vi "CastArrayDependenciesToClusterOrClass.vi"(7 "Dependency Type (Class|Cluster)":variant, 8 "error in (no error)":errorcluster, 10 "index (-1: from start)":i32=-1, 11 "[Dependencies]":refnum<class>[](array[class])) -> (0 "error out":errorcluster, 3 "Dependencies output":variant)   [LabVIEW 2019, in "SMO.lvclass"]
doc: "JKI State Machine Objects (SMO) 1.3.0.56\nJKI - JKI\nCopyright (c) 2017, JKI"
uses:
  SMO.lvclass
  <vilib>/Utility/VariantDataType/Type.ctl
  <vilib>/Utility/VariantDataType/VariantType.lvlib
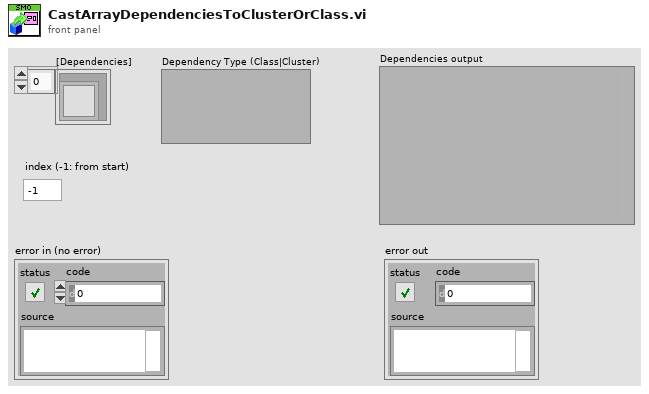
[diagram p1: front panel]
types:
  T1 = typedef "VariantType.lvlib/Type.ctl" = enum8{"Invalid Type", "Void", "I8", "I16", "I32", "I64", "U8", "U16", "U32", "U64", "Single Float", "Double Float", "Extended Float", "Single Complex", "Double Complex", "Extended Complex", "Enum U8", "Enum U16", "Enum U32", "Enum U64", "Single Float With Unit", "Double Float With Unit", "Extended Float With Unit", "Single Complex with Unit", "Double Complex with Unit", "Extended Complex with Unit", "Boolean", "String", "Path", "Picture", "Tag", "Array", "Cluster", "Variant", "LV Variant", "Waveform", "Timestamp", "Digital Waveform", "Digital Data", "ExpressData", "Refnum", "External Data", "VI", "Poly VI", "LabVIEW Class Instance", "Fixed Point"}
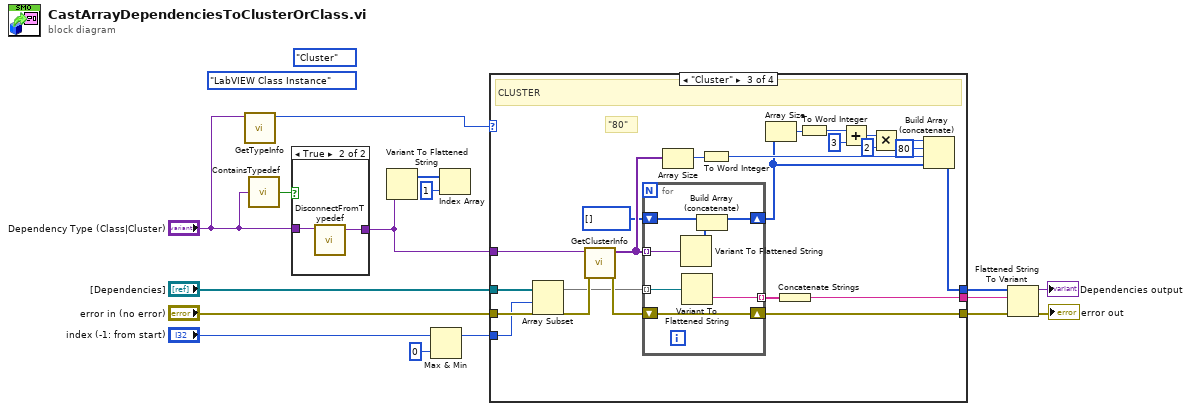
[diagram p0: block diagram]
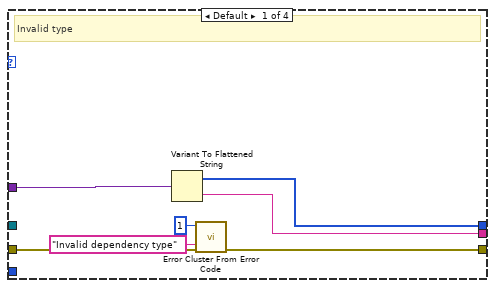
[diagram p3: hidden frame]
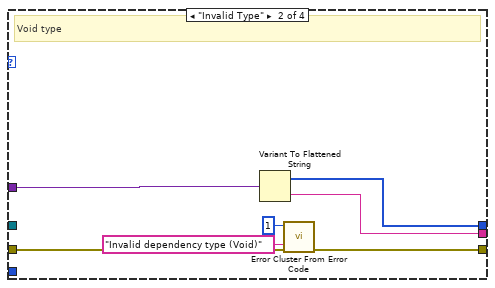
[diagram p4: hidden frame]
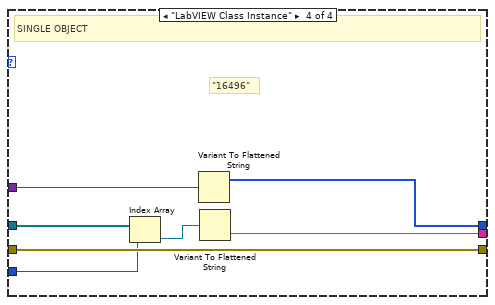
[diagram p5: hidden frame]
diagram:
  (unwired) Type."LabVIEW Class Instance" ("Type Enum")
  (unwired) Type."Cluster" ("Type Enum")
  n1 = call <vilib>:"GetTypeInfo.vi"("Variant"="Dependency Type (Class|Cluster)") -> ("Type Enum"=w1:T1)  [unwired: 6 in, 4 out]
  n2 = call <vilib>:"ContainsTypedef.vi"("lvvar"="Dependency Type (Class|Cluster)") -> ("Contains Typedef"=w4:bool)
  n3 = case shown="True" w4 {
    tunnel: "Dependency Type (Class|Cluster)" -> [w17 w19]
    tunnel: [w17 w18] -> w3
    frame False {
    }
    frame True {
      n4 = call <vilib>:"DisconnectFromTypedef.vi"("lvvar in"=w19) -> ("lvvar out"=w18:variant)  [unwired: 4 in, 1 out]
    }
  }
  n5 = Variant To Flattened String(Variant=w3) -> (1:w9:i16[])  [unwired: 1 out]
  n6 = Max & Min(x="index (-1: from start)", y=0) -> (max(x,y)=w5:i32)  [unwired: 1 out]
  n7 = Index Array(array=w9, index=1) -> ()  [unwired: 1 out]
  n8 = case shown="\"Cluster\"" w1 {
    tunnel: [w22 w29 w55 w68] -> w14
    tunnel: "[Dependencies]" -> [_ _ w36 w65]
    tunnel: "error in (no error)" -> [w23 w30 w54 w68]
    tunnel: [w24 w31 w47 w66] -> w11
    tunnel: [w25 w32 w39 w67] -> w10
    tunnel: w3 -> [w26 w33 w38 w69]
    tunnel: w5 -> [_ _ w34 w63]
    frame Default {
      # "Invalid type"
      n9 = Variant To Flattened String(Variant=w26) -> (data string=w24:string, 1:w25:i16[])
      n10 = call <vilib>:"Error Cluster From Error Code.vi"("error in (no error)"=w23, "error message (\"\")"="Invalid dependency type" ("error message (\"\")"), "error code (0)"=1) -> ("error out"=w22:errorcluster)  [unwired: 6 in]
    }
    frame "Invalid Type" {
      # "Void type"
      n11 = Variant To Flattened String(Variant=w33) -> (data string=w31:string, 1:w32:i16[])
      n12 = call <vilib>:"Error Cluster From Error Code.vi"("error in (no error)"=w30, "error message (\"\")"="Invalid dependency type (Void)" ("error message (\"\")"), "error code (0)"=1) -> ("error out"=w29:errorcluster)  [unwired: 6 in]
    }
    frame "Cluster" {
      # "\"80\""
      # "CLUSTER"
      n13 = Array Subset(array=w36, index=w34) -> (w35:refnum<class>[])  [unwired: 1 in]
      n14 = call <vilib>:"GetClusterInfo.vi"("error in (no error)"=w54, "Variant"=w38) -> ("error out"=w53:errorcluster, "Cluster Elements"=w52:variant[])  [unwired: 8 in]
      n15 = for {
        tunnel: w35 -> [w62] mode=indexing
        shift-right: [w61] -> w55
        shift-left: w53 -> [w61]
        tunnel: w52 -> [w60] mode=indexing
        shift-right: [w58] -> w40
        shift-left: i16[] [] -> [w59]
        tunnel: [w57] -> w48 mode=indexing
        n16 = Variant To Flattened String(Variant=w60) -> (1:w56:i16[])  [unwired: 1 out]
        n17 = Variant To Flattened String(Variant=w62) -> (data string=w57:string)  [unwired: 1 out]
        n18 = Build Array (concatenate)(w59, w56) -> (w58:i16[])
      }
      n19 = Array Size(array=w52) -> (size(s)=w51:i32)
      n20 = To Word Integer(number=w51) -> (16bit integer=w50:i16)
      n21 = Array Size(array=w40) -> (size(s)=w42:i32)
      n22 = Concatenate Strings(w48) -> (w47:string)
      n23 = To Word Integer(number=w42) -> (16bit integer=w46:i16)
      n24 = Add(x=w46, y=i16 3) -> (x+y=w44:i16)
      n25 = Multiply(x=w44, y=i16 2) -> (x*y=w41:i16)
      n26 = Build Array (concatenate)(w41, i16 80 ("16bit integer"), w50, w40) -> (w39:i16[])
    }
    frame "LabVIEW Class Instance" {
      # "\"16496\""
      # "SINGLE OBJECT"
      n27 = Index Array(array=w65, index=w63) -> (element=w64:refnum<class>)
      n28 = Variant To Flattened String(Variant=w69) -> (1:w67:i16[])  [unwired: 1 out]
      n29 = Variant To Flattened String(Variant=w64) -> (data string=w66:string)  [unwired: 1 out]
    }
  }
  n30 = Flattened String To Variant(4:w14, 6:w11, 7:w10) -> (0:→"error out":errorcluster, 3:→"Dependencies output":variant)
